vi "cDAQ Channel Tester.vi"(8 "error in (no error)":errorcluster) -> (0 "error out":errorcluster)   [LabVIEW 2016]
uses:
  <resource>/objmgr/daqmx.rc
panel:
  in  "Scan Rate (mSec)":i32=1000
  out "cDAQ Data":string[][](array[string])
  in  "Tab Control":enum32{"Settings"}(tab)
  in  "Tasks In":refnum<k21>[](array[refnum])=["TC Temps-Module 1", "TC Temps-Module 2", "TC Temps-Module 3", "TC Temps-Module 4", "TC Temps-Module 5", "Gas and Temp-Module 6", "AC_DC Events-Module 7"]
  in  "Debug":bool
  out "Debug Data":string[](array[string])
  in  "EXIT":bool
  # "NI DAQ Channel Tester"
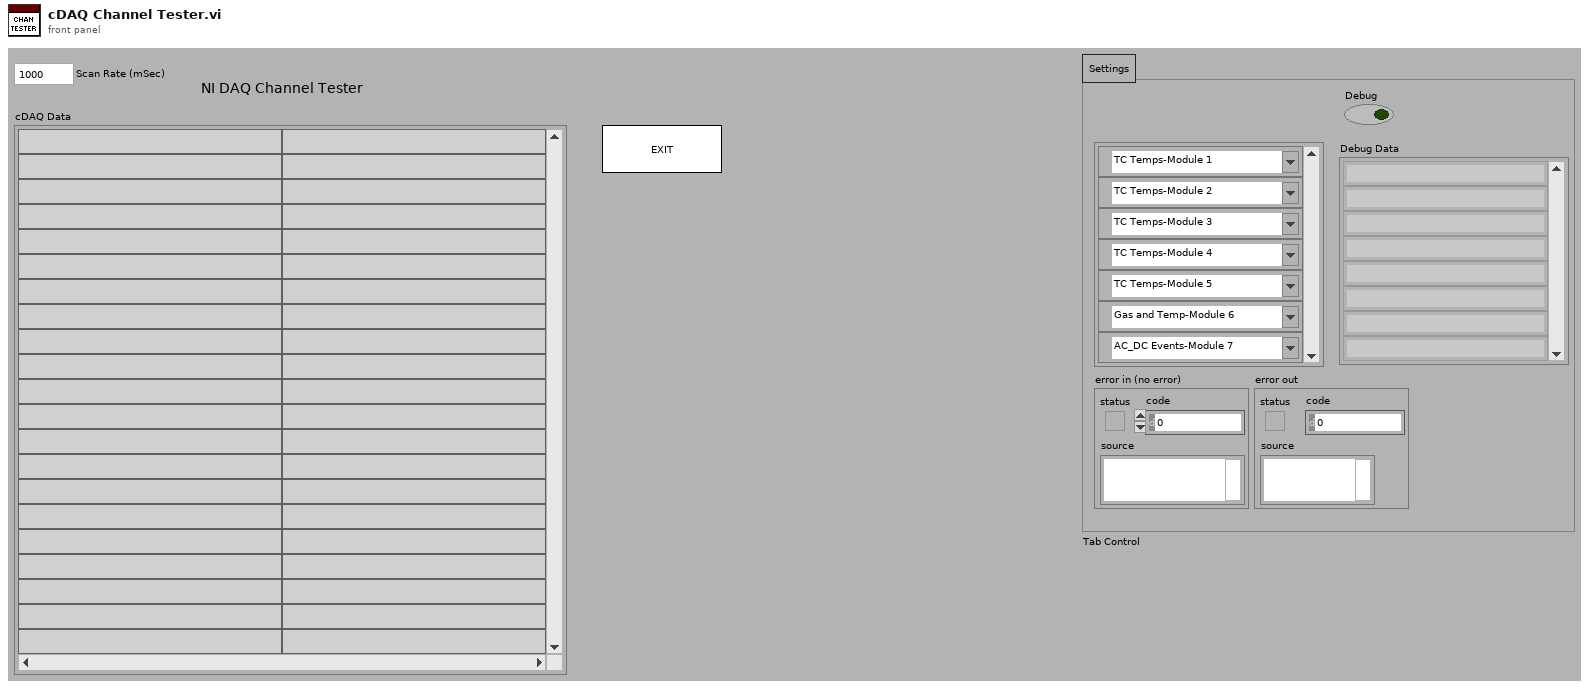
[diagram p1: front panel]
types:
  T1 = enum32{"invalid app kind", "Development System", "Run Time System", "Student Edition", "Embedded LabVIEW", "Evaluation", "Custom"}
  T2 = enum32{"Invalid", "Standard", "Closed", "Hidden", "Minimized", "Maximized"}
  T3 = cluster{"Core":cluster{"Current VI Reference":refnum<vi>, "Close Panel on Exit?":bool}, "Tasks In":refnum<k21>[]}
  T4 = cluster{"Current VI Reference":refnum<vi>, "Close Panel on Exit?":bool}
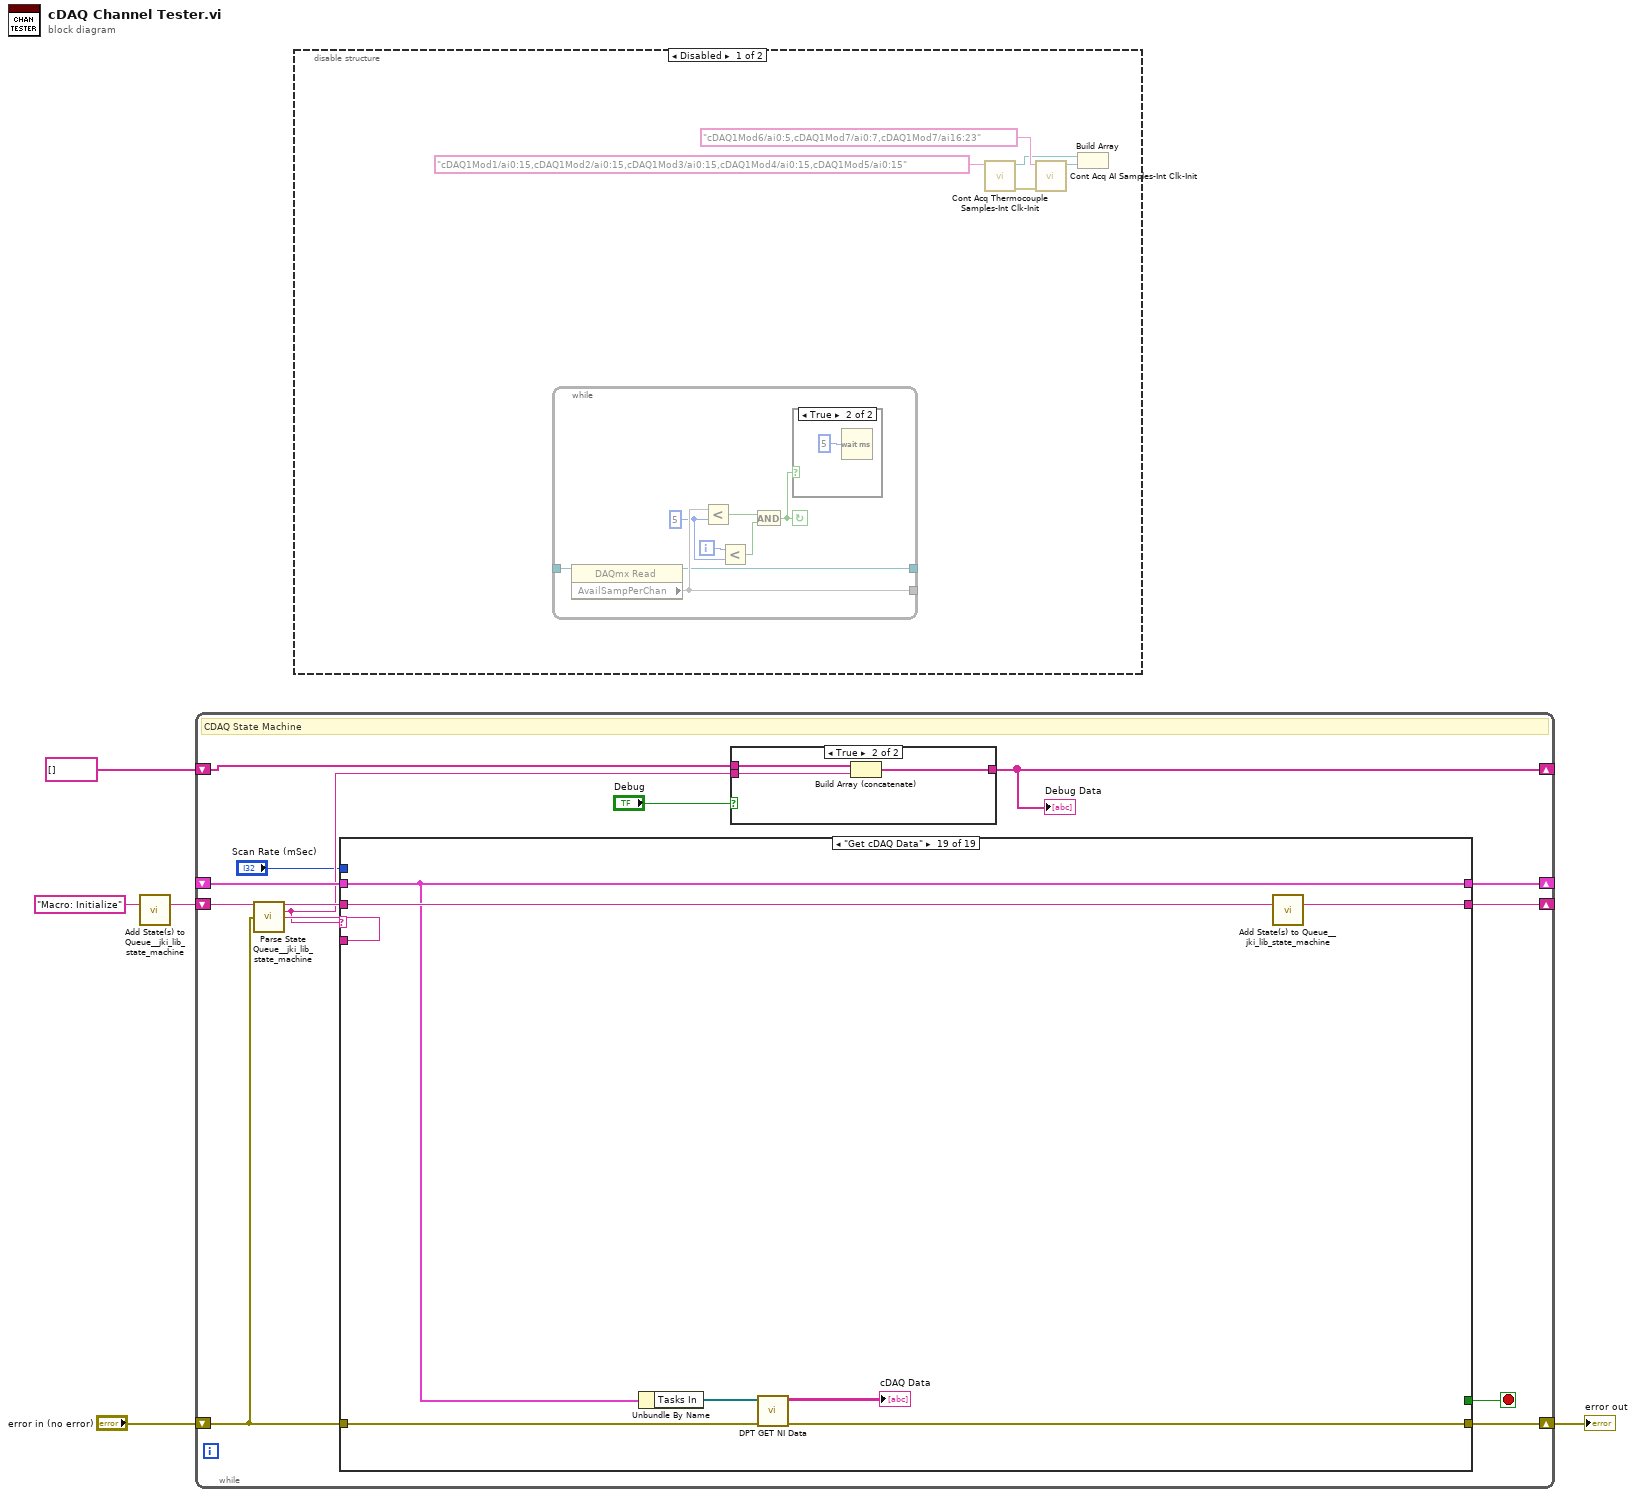
[diagram p0: block diagram]
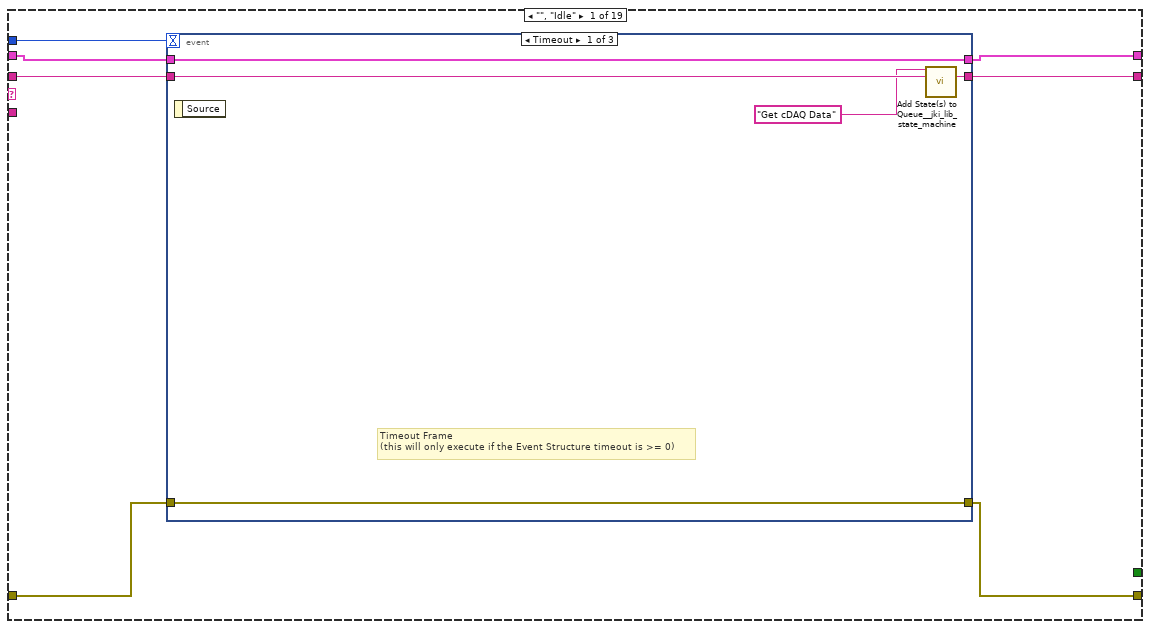
[diagram p5: hidden frame]
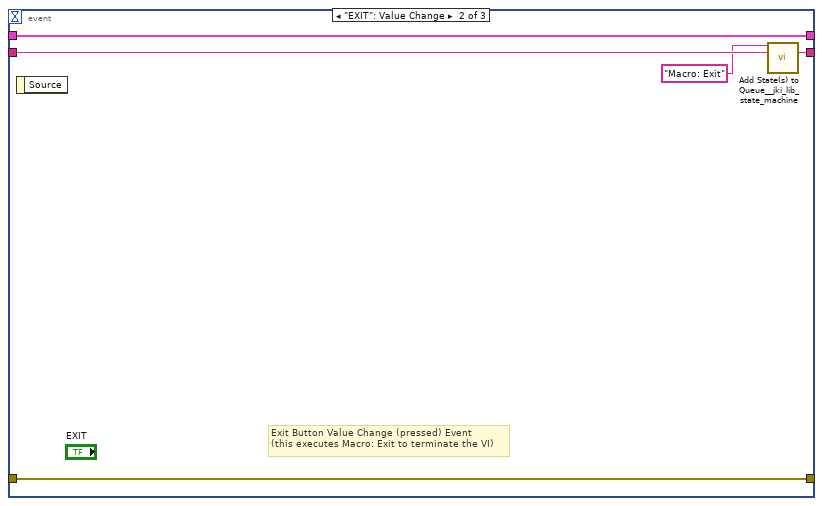
[diagram p6: hidden frame]
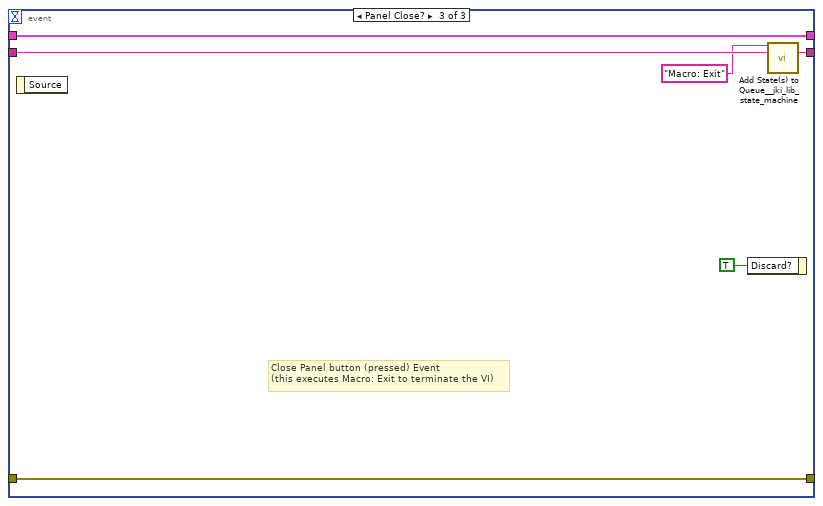
[diagram p7: hidden frame]
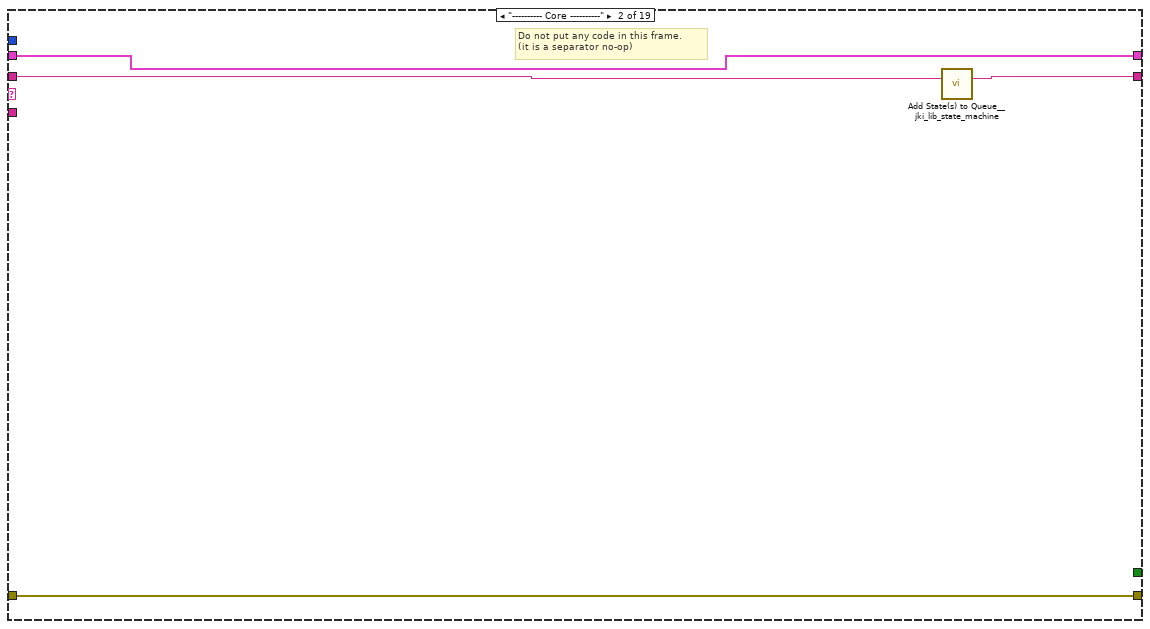
[diagram p8: hidden frame]
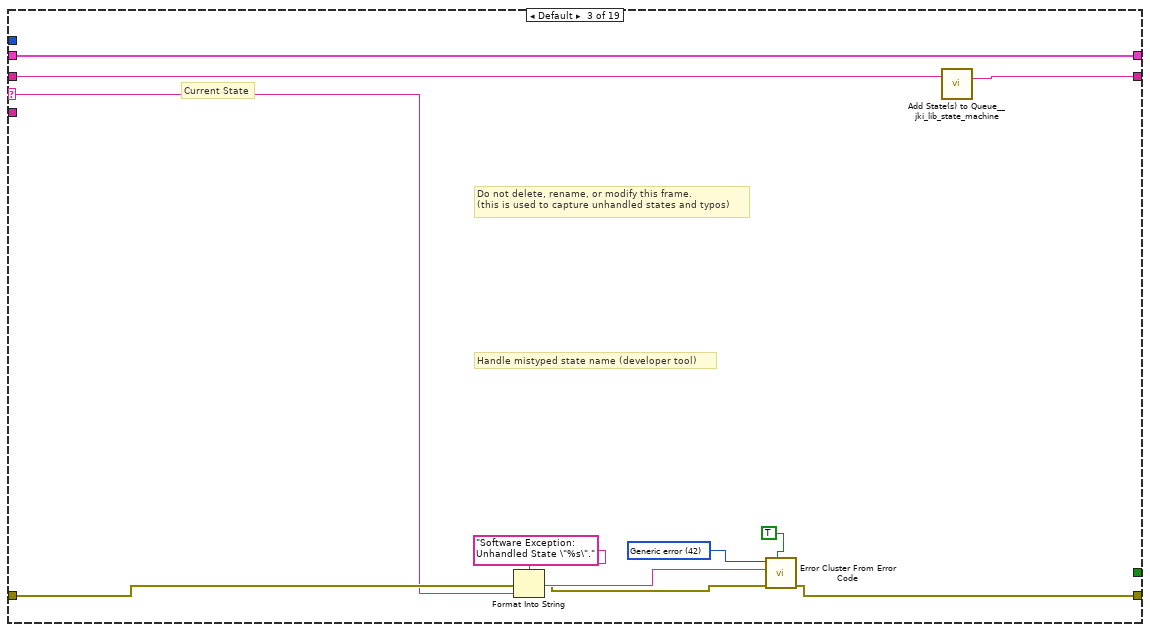
[diagram p9: hidden frame]
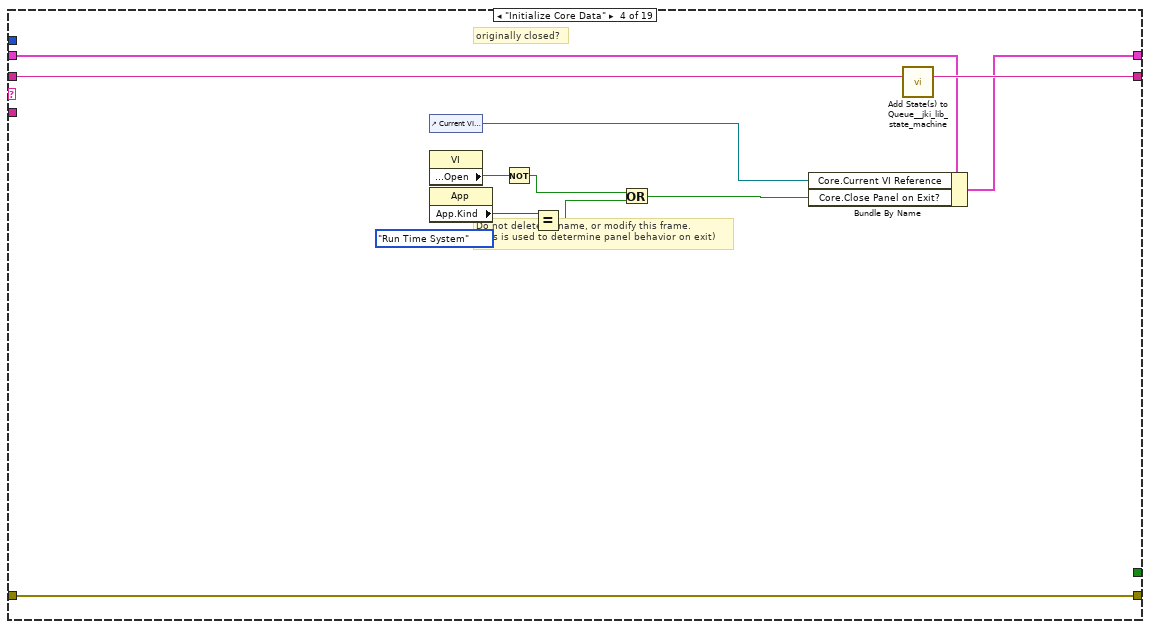
[diagram p10: hidden frame]
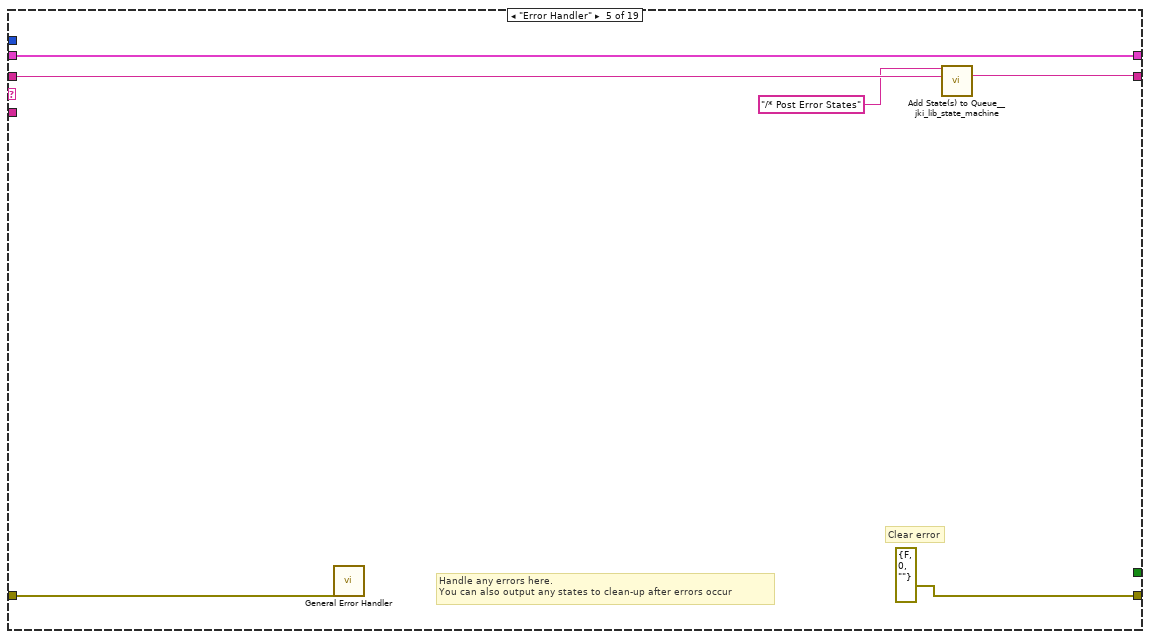
[diagram p11: hidden frame]
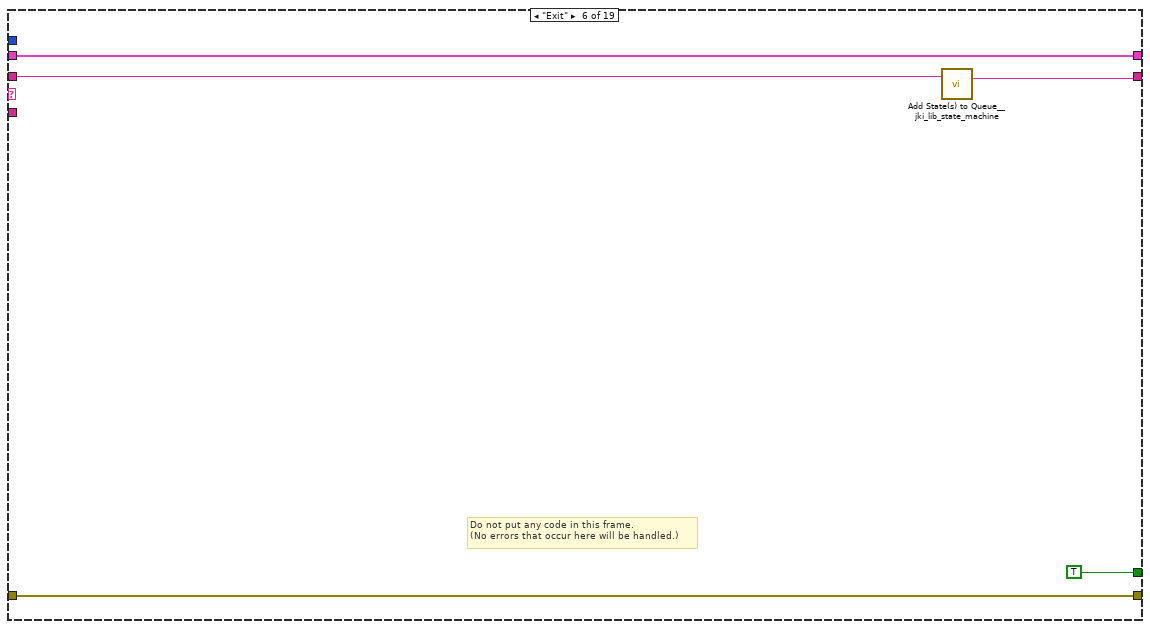
[diagram p12: hidden frame]
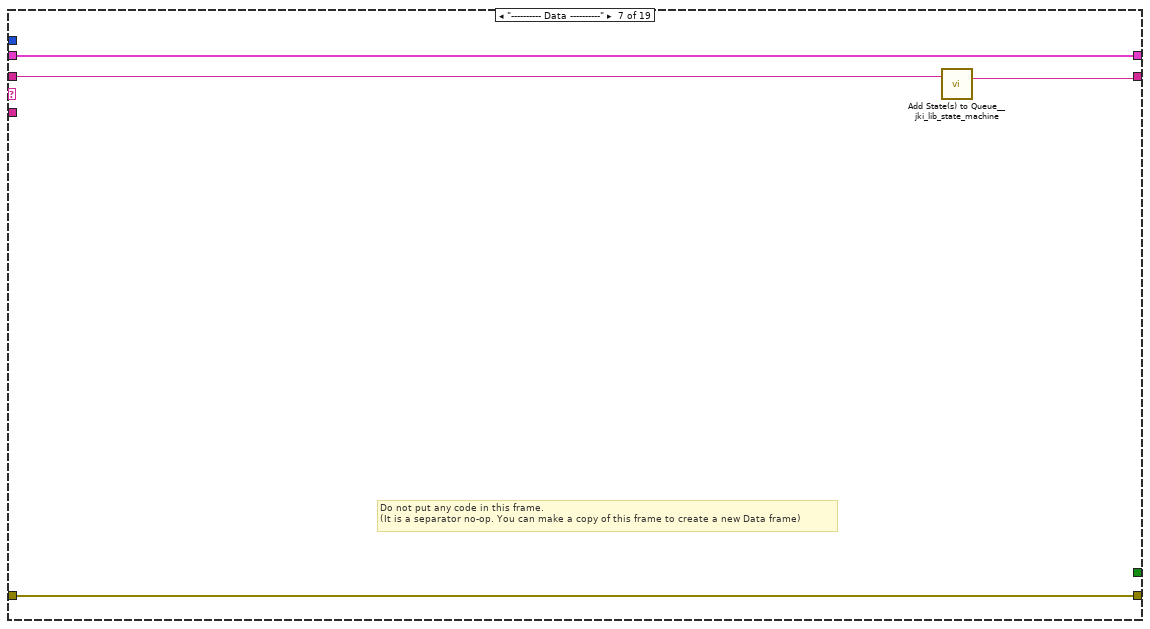
[diagram p13: hidden frame]
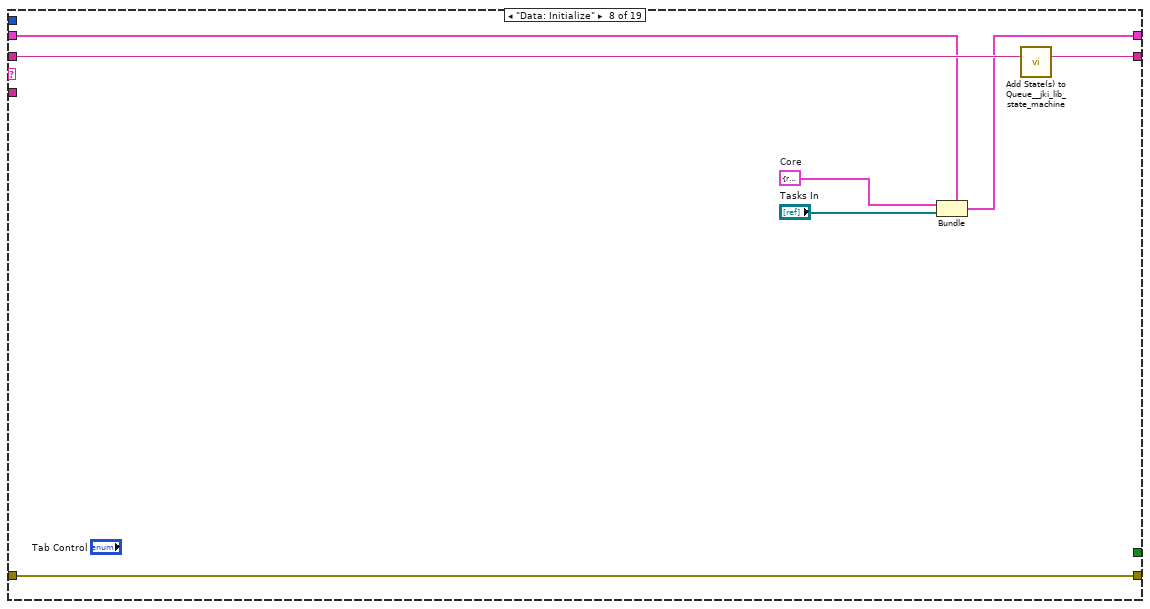
[diagram p14: hidden frame]
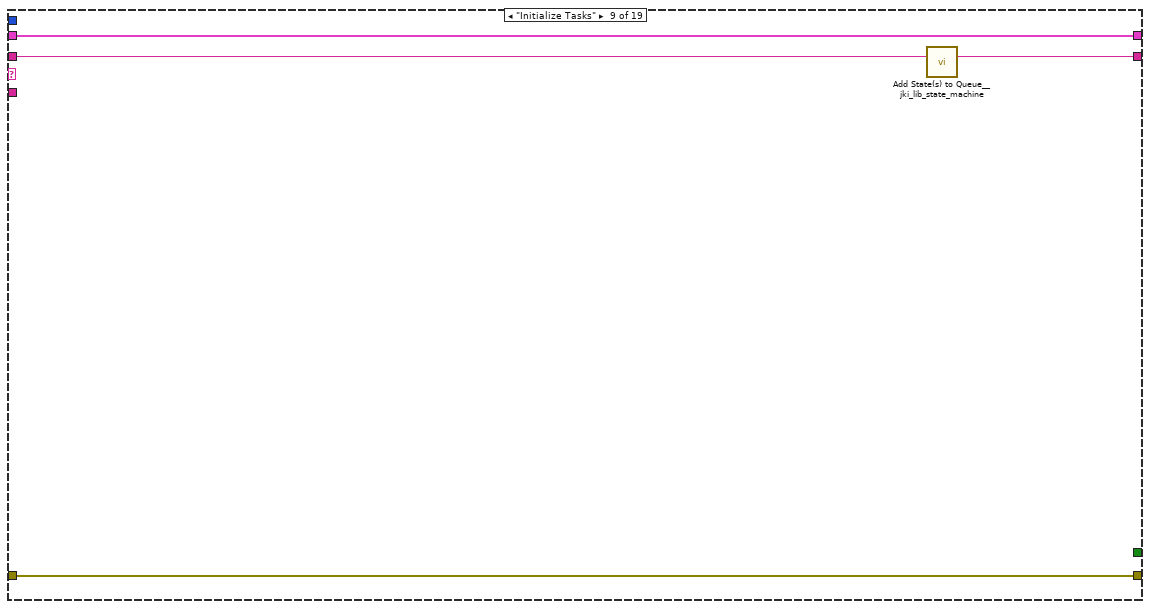
[diagram p15: hidden frame]
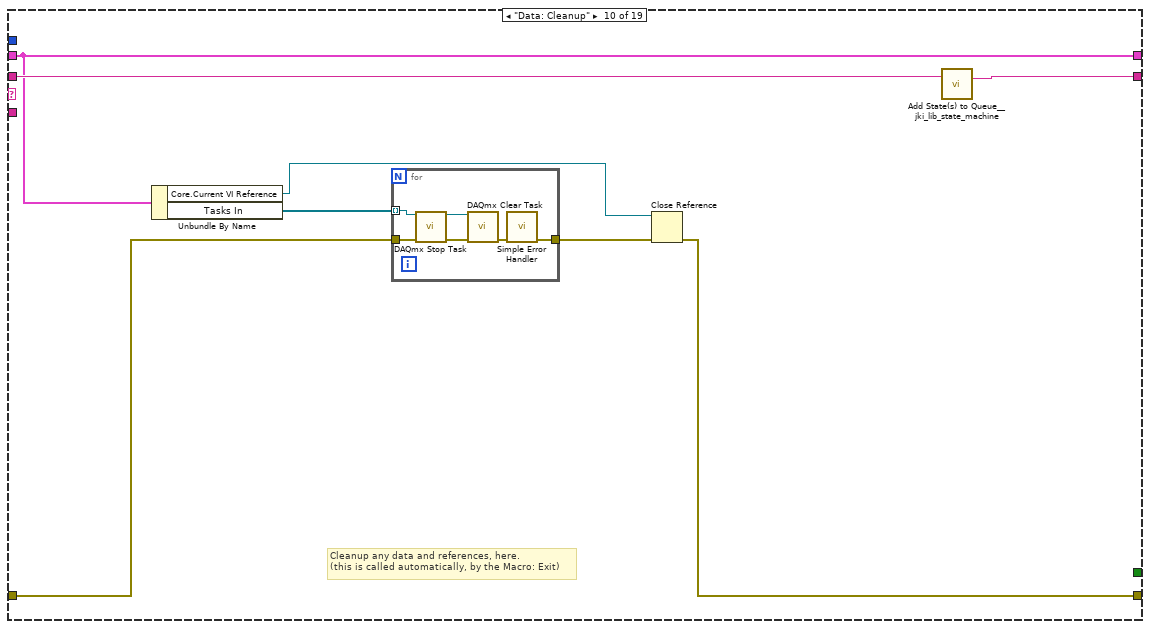
[diagram p16: hidden frame]
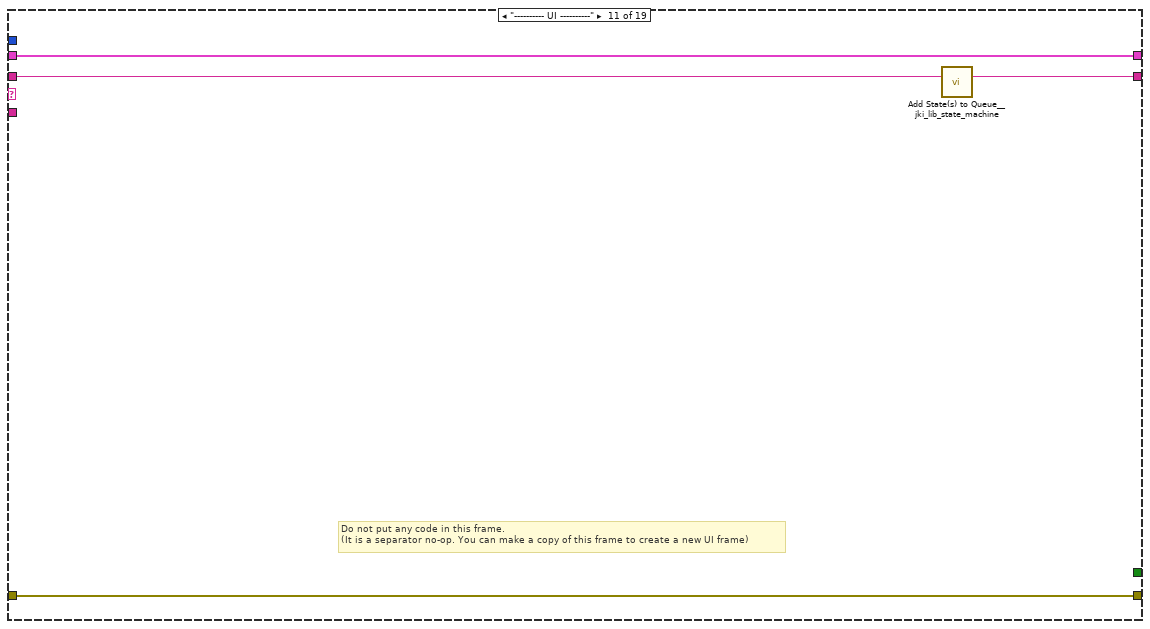
[diagram p17: hidden frame]
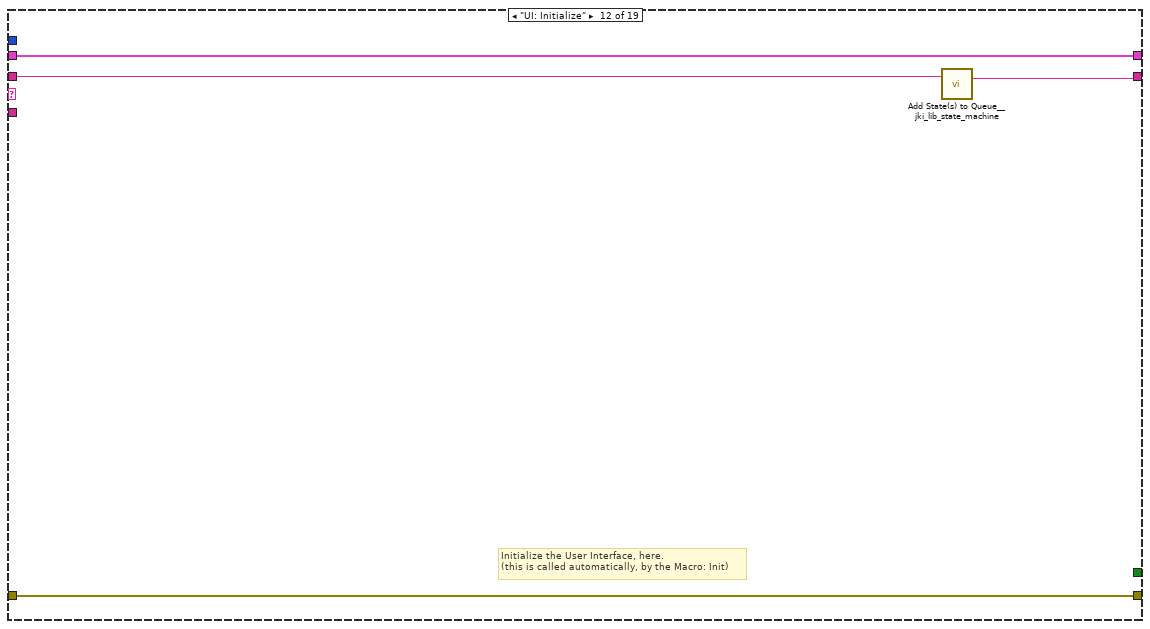
[diagram p18: hidden frame]
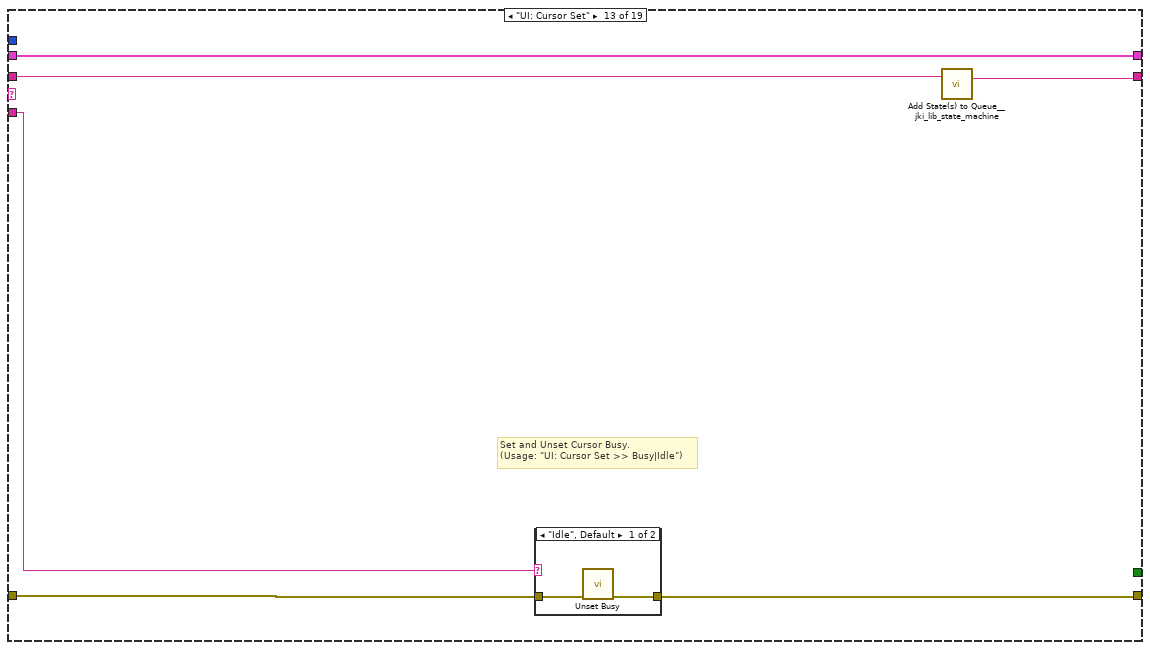
[diagram p19: hidden frame]
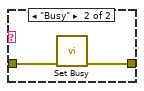
[diagram p20: hidden frame]
diagram:
  n1 = call <vilib>:"Add State(s) to Queue__jki_lib_state_machine.vi"("State(s) in (\"\")"="Macro: Initialize") -> ("States Out"=w5:string)  [unwired: 14 in]
  n2 = while "CDAQ State Machine" {
    shift-right: [w14] -> _
    shift-left: _ -> [w13]
    shift-right: [w16] -> w2
    shift-left: "error in (no error)" -> [w12]
    shift-right: [w15] -> _
    shift-left: w5 -> [w17]
    shift-right: [w9] -> _
    shift-left: string[] [] -> [w10]
    stop <- w11 stop-if-true
    # "CDAQ State Machine"
    n3 = call <vilib>:"Parse State Queue__jki_lib_state_machine.vi"("State Queue"=w17, "Error In (no error)"=w12) -> ("Remaining States"=w19:string, "Current State"=w8:string, "Arguments"=w18:string)  [unwired: 11 in]
    n4 = case shown="\"Get cDAQ Data\"" w8 {
      selector: w8 -> [_ _ w51 _ _ _ _ _ _ _ _ _ _ _ _ _ _ _ _]
      tunnel: w19 -> [w30 w50 w55 w73 w79 w84 w88 w95 w99 w107 w117 w121 w127 w138 w164 w169 w179 w183 w190]
      tunnel: w18 -> [_ _ _ _ _ _ _ _ _ _ _ _ w122 w132 _ _ _ _ _]
      tunnel: w13 -> [w28 w47 w53 w64 w75 w82 w85 w90 w97 w104 w114 w119 w125 w134 w161 w166 w176 w180 w185]
      tunnel: [w27 w48 w57 w70 errorcluster {"status"=FALSE, "code"=0, "source"=""} ("error out") w81 w86 w91 w96 w105 w115 w118 w123 w135 w162 w167 w177 w181 w187] -> w16
      tunnel: w12 -> [w26 w48 w56 w70 w74 w81 w86 w91 w96 w103 w115 w118 w124 w136 w162 w167 w177 w181 w188]
      tunnel: [w29 w49 w54 w72 w78 w83 w87 w94 w98 w106 w116 w120 w126 w137 w163 w168 w178 w182 w189] -> w15
      tunnel: [_ _ _ _ _ TRUE _ _ _ _ _ _ _ _ _ _ _ _ _] -> w11
      tunnel: [w25 w47 w53 w71 w75 w82 w85 w93 w97 w104 w114 w119 w125 w134 w161 w166 w176 w180 w185] -> w14
      tunnel: "Scan Rate (mSec)" -> [w24 _ _ _ _ _ _ _ _ _ _ _ _ _ _ _ _ _ _]
      frame "", "Idle" {
        n5 = event shown="[0] Timeout" {
          selector: _ -> [_ _ _]
          dyn-events: _ -> [_ _ _]
          timeout: w24 -> [_ _ _]
          tunnel: w30 -> [w35 w40 w46]
          tunnel: [w34 w39 w45] -> w29
          tunnel: w28 -> [w32 w37 w43]
          tunnel: [w33 w38 w44] -> w27
          tunnel: w26 -> [w33 w38 w44]
          tunnel: [w32 w37 w43] -> w25
          event Timeout {
            # "Timeout Frame\n(this will only execute if the Event Structure timeout is >= 0)"
            n6 = event-data() -> ()  [unwired: 1 in, 1 out]
            n7 = call <vilib>:"Add State(s) to Queue__jki_lib_state_machine.vi"("State(s) in Front (\"\")"="Get cDAQ Data", "State(s) in (\"\")"=w35) -> ("States Out"=w34:string)  [unwired: 13 in]
          }
          event "EXIT": Value Change {
            # "Exit Button Value Change (pressed) Event\n(this executes Macro: Exit to terminate the VI)"
            n8 = event-data() -> ()  [unwired: 1 in, 1 out]
            n9 = call <vilib>:"Add State(s) to Queue__jki_lib_state_machine.vi"("State(s) in Front (\"\")"="Macro: Exit", "State(s) in (\"\")"=w40) -> ("States Out"=w39:string)  [unwired: 13 in]
          }
          event Panel Close? {
            # "Close Panel button (pressed) Event\n(this executes Macro: Exit to terminate the VI)"
            n10 = event-data() -> ()  [unwired: 1 in, 1 out]
            n11 = event-data("Discard?"=TRUE) -> ()  [unwired: 1 in, 1 out]
            n12 = call <vilib>:"Add State(s) to Queue__jki_lib_state_machine.vi"("State(s) in Front (\"\")"="Macro: Exit", "State(s) in (\"\")"=w46) -> ("States Out"=w45:string)  [unwired: 13 in]
          }
        }
      }
      frame "---------- Core ----------" {
        # "Do not put any code in this frame.\n(it is a separator no-op)"
        n13 = call <vilib>:"Add State(s) to Queue__jki_lib_state_machine.vi"("State(s) in (\"\")"=w50) -> ("States Out"=w49:string)  [unwired: 14 in]
      }
      frame Default {
        w60 = 42 items=["No error", "Argument error", "Memory is full", "Out of zone", "End of file", "File already open", "Generic file I/O error", "File not found", "File permission error", "Disk is full", "Duplicate path", "Too many files open", "System feature not enabled", "Resource file not found", "Cannot add resource", "Resource not found", "Image not found", "Image memory error", "Pen does not exist", "Config type invalid", "Config token not found", "Config parse error", "Config memory error", "Bad external code format", "Bad external code offset", "External code not present", "Null window", "Destroy window error", "Null menu", "Print aborted", "Bad print record", "Print driver error", "Windows error during printing", "Memory error during printing", "Print dialog error", "Generic print error", "Invalid device refnum", "Device not found", "Device parameter error", "Device unit error", "Cannot open device", "Device call aborted", "Generic error", "Cancelled by user", "Object ID too low", "Object ID too high", "Object not in heap", "Unknown heap", "Unknown object (invalid DefProc)", "Unknown object (DefProc not in table)", "Message out of range", "Invalid (null) method", "Unknown message", "Manager call not supported", "Bad address", "Network operation in progress", "Network operation timed out", "Connection is busy", "Network attribute not supported", "Network error", "Address in use", "System out of memory", "Connection aborted", "Connection refused", "Not connected", "Already connected", "Connection closed", "Initialization error (interapplication manager)", "Bad occurrence", "Wait on unbound occurrence handler", "Occurrence queue overflow", "Datalog type conflict", "Unused", "Unrecognized type (interapplication manager)", "Memory corrupt", "Failed to make temporary DLL", "Old CIN version", "Drag socket not found", "Failed to load drop-object", "Failed to register OLE object", "Failed to release OLE object", "Format specifier type mismatch", "Unknown format specifier", "Too few format specifiers", "Too many format specifiers", "Scan failed", "Newer CIN version", "Error converting to variant", "Runtime menu error", "Password tampered", "Variant attribute not found", "Incompatible variant data type", "Event data is not available", "Event Store is not present", "Occurrence is not found", "Event Queue is not created", "Event info is not available", "Refnum passed is NULL", "Error retrieving Class GUID", "Error retrieving CoClass GUID", "Error retrieving TypeLib GUID.", "Bad built application magic bytes.", "Specific driver is different from the specific driver associated with the Logical Name.", "There is no session opened to the class driver.", "Max Error", "MAX - Error with config objects", "MAX - Error loading configuration", "MAX - Group not supported"]
        # "Current State"
        # "Do not delete, rename, or modify this frame.\n(this is used to capture unhandled states and typos)"
        # "Handle mistyped state name (developer tool)"
        n14 = Format Into String(format string="Software Exception: Unhandled State \"%s\"." ("message"), error in=w56, w51) -> (resulting string=w59:string, error out=w58:errorcluster)  [unwired: 1 in]
        n15 = call <vilib>:"Error Cluster From Error Code.vi"("show call chain? (False)"=TRUE, "error in (no error)"=w58, "error message (\"\")"=w59, "error code (0)"=w60) -> ("error out"=w57:errorcluster)  [unwired: 5 in]
        n16 = call <vilib>:"Add State(s) to Queue__jki_lib_state_machine.vi"("State(s) in (\"\")"=w55) -> ("States Out"=w54:string)  [unwired: 14 in]
      }
      frame "Initialize Core Data" {
        # "Do not delete, rename, or modify this frame.\n(this is used to determine panel behavior on exit)"
        # "originally closed?"
        n17 = control-ref of="Current VI Reference"() -> (w62:refnum<vi>)
        n18 = property class="VI"() -> ("Front Panel.Open"=w69:bool)  [unwired: 2 in, 2 out]
        n19 = property class="App"() -> ("App.Kind"=w68:T1)  [unwired: 2 in, 2 out]
        n20 = Not(x=w69) -> (.not. x?=w66:bool)
        n21 = Equal?(x=w68, y=T1."Run Time System" ("Application:Kind")) -> (x = y?=w65:bool)
        n22 = Or(x=w66, y=w65) -> (x .or. y?=w63:bool)
        n23 = Bundle By Name(cluster=w64, "Core.Current VI Reference"=w62, "Core.Close Panel on Exit?"=w63) -> (w71:T3)
        n24 = call <vilib>:"Add State(s) to Queue__jki_lib_state_machine.vi"("State(s) in (\"\")"=w73) -> ("States Out"=w72:string)  [unwired: 14 in]
      }
      frame "Error Handler" {
        # "Handle any errors here.\nYou can also output any states to clean-up after errors occur"
        # "Clear error"
        n25 = call <vilib>:"General Error Handler.vi"("error in (no error)"=w74) -> ()  [unwired: 10 in, 5 out]
        n26 = call <vilib>:"Add State(s) to Queue__jki_lib_state_machine.vi"("State(s) in Front (\"\")"="/* Post Error States", "State(s) in (\"\")"=w79) -> ("States Out"=w78:string)  [unwired: 13 in]
      }
      frame "Exit" {
        # "Do not put any code in this frame.\n(No errors that occur here will be handled.)"
        n27 = call <vilib>:"Add State(s) to Queue__jki_lib_state_machine.vi"("State(s) in (\"\")"=w84) -> ("States Out"=w83:string)  [unwired: 14 in]
      }
      frame "---------- Data ----------" {
        # "Do not put any code in this frame.\n(It is a separator no-op. You can make a copy of this frame to create a new Data frame)"
        n28 = call <vilib>:"Add State(s) to Queue__jki_lib_state_machine.vi"("State(s) in (\"\")"=w88) -> ("States Out"=w87:string)  [unwired: 14 in]
      }
      frame "Data: Initialize" {
        w92 = T4 {"Current VI Reference"=refnum, "Close Panel on Exit?"=FALSE}  # Core
        n29 = Bundle(cluster=w90, "Core"=w92, "Tasks In"="Tasks In") -> (w93:T3)
        n30 = call <vilib>:"Add State(s) to Queue__jki_lib_state_machine.vi"("State(s) in (\"\")"=w95) -> ("States Out"=w94:string)  [unwired: 14 in]
      }
      frame "Initialize Tasks" {
        n31 = call <vilib>:"Add State(s) to Queue__jki_lib_state_machine.vi"("State(s) in (\"\")"=w99) -> ("States Out"=w98:string)  [unwired: 14 in]
      }
      frame "Data: Cleanup" {
        # "Cleanup any data and references, here.\n(this is called automatically, by the Macro: Exit)"
        n32 = Unbundle By Name(w104) -> ("Core.Current VI Reference"=w101:refnum<vi>, "Tasks In"=w100:refnum<k21>[])
        n33 = for {
          tunnel: w103 -> [w112]
          tunnel: [w108] -> w102
          tunnel: w100 -> [w109] mode=indexing
          n34 = call <vilib>:"DAQmx Stop Task.vi"("task/channels in"=w109, "error in"=w112) -> ("task out"=w110:refnum<k21>, "error out"=w111:errorcluster)  [unwired: 12 in]
          n35 = call <vilib>:"DAQmx Clear Task.vi"("task in"=w110, "error in"=w111) -> ("error out"=w113:errorcluster)  [unwired: 13 in]
          n36 = call <vilib>:"Simple Error Handler.vi"("error in (no error)"=w113) -> ("error out"=w108:errorcluster)  [unwired: 4 in, 4 out]
        }
        n37 = Close Reference(reference=w101, error in (no error)=w102) -> (error out=w105:errorcluster)
        n38 = call <vilib>:"Add State(s) to Queue__jki_lib_state_machine.vi"("State(s) in (\"\")"=w107) -> ("States Out"=w106:string)  [unwired: 14 in]
      }
      frame "---------- UI ----------" {
        # "Do not put any code in this frame.\n(It is a separator no-op. You can make a copy of this frame to create a new UI frame)"
        n39 = call <vilib>:"Add State(s) to Queue__jki_lib_state_machine.vi"("State(s) in (\"\")"=w117) -> ("States Out"=w116:string)  [unwired: 14 in]
      }
      frame "UI: Initialize" {
        # "Initialize the User Interface, here.\n(this is called automatically, by the Macro: Init)"
        n40 = call <vilib>:"Add State(s) to Queue__jki_lib_state_machine.vi"("State(s) in (\"\")"=w121) -> ("States Out"=w120:string)  [unwired: 14 in]
      }
      frame "UI: Cursor Set" {
        # "Set and Unset Cursor Busy.\n(Usage: \"UI: Cursor Set >> Busy|Idle\")"
        n41 = case shown="\"Idle\", Default" w122 {
          tunnel: w124 -> [w129 w131]
          tunnel: [w128 w130] -> w123
          frame "Idle", Default {
            n42 = call <vilib>:"Unset Busy.vi"("error in (no error)"=w129) -> ("error out"=w128:errorcluster)  [unwired: 10 in]
          }
          frame "Busy" {
            n43 = call <vilib>:"Set Busy.vi"("error in (no error)"=w131) -> ("error out"=w130:errorcluster)  [unwired: 9 in, 1 out]
          }
        }
        n44 = call <vilib>:"Add State(s) to Queue__jki_lib_state_machine.vi"("State(s) in (\"\")"=w127) -> ("States Out"=w126:string)  [unwired: 14 in]
      }
      frame "UI: Front Panel State" {
        # "Argument"
        # "Set Front Panel Open or Closed\n(Usage: \"UI: Front Panel State >> Open|Close\")"
        n45 = Unbundle By Name(w134) -> ("Core.Current VI Reference"=w133:refnum<vi>)
        n46 = case shown="\"Close\"" w132 {
          tunnel: w136 -> [w142 w155]
          tunnel: [w144 w156] -> w135
          tunnel: w133 -> [w143 w153]
          frame "Open", Default {
            n47 = property class="VI"(reference=w143, error in=w142) -> (reference out=w140:refnum<vi>, error out=w141:errorcluster, "Front Panel.Open"=w139:bool)
            n48 = case shown="False" w139 {
              tunnel: [w147 w150] -> w144
              tunnel: w141 -> [w146 w150]
              tunnel: w140 -> [w145 _]
              frame False {
                n49 = invoke class="VI" method="FP.Open"(reference=w145, error in=w146, "Activate"=TRUE, "State"=T2."Standard") -> (error out=w147:errorcluster)  [unwired: 1 in, 4 out]
              }
              frame True {
              }
            }
          }
          frame "Close" {
            n50 = property class="VI"(reference=w153, error in=w155) -> (reference out=w152:refnum<vi>, error out=w154:errorcluster, "Front Panel.Open"=w151:bool)
            n51 = case shown="True" w151 {
              tunnel: [w157 w160] -> w156
              tunnel: w154 -> [w157 w159]
              tunnel: w152 -> [_ w158]
              frame False {
              }
              frame True {
                n52 = invoke class="VI" method="FP.Close"(reference=w158, error in=w159) -> (error out=w160:errorcluster)  [unwired: 1 in, 2 out]
              }
            }
          }
        }
        n53 = call <vilib>:"Add State(s) to Queue__jki_lib_state_machine.vi"("State(s) in (\"\")"=w138) -> ("States Out"=w137:string)  [unwired: 14 in]
      }
      frame "---------- Macro ----------" {
        # "Do not put any code in this frame.\n(It is a separator no-op. You can make a copy of this frame to create a new Macro frame)"
        n54 = call <vilib>:"Add State(s) to Queue__jki_lib_state_machine.vi"("State(s) in (\"\")"=w164) -> ("States Out"=w163:string)  [unwired: 14 in]
      }
      frame "Macro: Initialize" {
        # "Initialization Macro\n(This is called once, when the VI starts)"
        n55 = call <vilib>:"Add State(s) to Queue__jki_lib_state_machine.vi"("State(s) in Front (\"\")"="Data: Initialize\nInitialize Core Data\nUI: Initialize\nUI: Front Panel State >> Open", "State(s) in (\"\")"=w169) -> ("States Out"=w168:string)  [unwired: 13 in]
      }
      frame "Macro: Exit" {
        # "Exit Macro\n(This is called once, when the VI exits)"
        n56 = Unbundle By Name(w176) -> ("Core.Close Panel on Exit?"=w175:bool)
        n57 = Select(t="UI: Front Panel State >> Close", s=w175, f="") -> (s? t:f=w172:string)
        n58 = call <vilib>:"Add State(s) to Queue__jki_lib_state_machine.vi"("State(s) in (\"\")"=w172, "State(s) at Back (\"\")"="Data: Cleanup\nExit") -> ("States Out"=w170:string)  [unwired: 13 in]
        n59 = call <vilib>:"Add State(s) to Queue__jki_lib_state_machine.vi"("State(s) in Front (\"\")"=w170, "State(s) in (\"\")"=w179) -> ("States Out"=w178:string)  [unwired: 13 in]
      }
      frame "------ TestDAQ ------" {
        # "Template Separator\n(You can make a copy of, or modify, this frame)"
        n60 = call <vilib>:"Add State(s) to Queue__jki_lib_state_machine.vi"("State(s) in (\"\")"=w183) -> ("States Out"=w182:string)  [unwired: 14 in]
      }
      frame "Get cDAQ Data" {
        n61 = Unbundle By Name(w185) -> ("Tasks In"=w184:refnum<k21>[])
        n62 = call "DPT GET NI Data.vi"("error in (no error)"=w188, "Tasks In"=w184) -> ("error out"=w187:errorcluster, "cDAQ Data"=→"cDAQ Data":string[][])  [unwired: 7 in, 1 out]
        n63 = call <vilib>:"Add State(s) to Queue__jki_lib_state_machine.vi"("State(s) in (\"\")"=w190) -> ("States Out"=w189:string)  [unwired: 14 in]
      }
    }
    n64 = case shown="True" "Debug" {
      tunnel: w10 -> [w20 w23]
      tunnel: [w20 w22] -> w9
      tunnel: w8 -> [_ w21]
      frame False {
      }
      frame True {
        n65 = Build Array (concatenate)(w23, w21) -> (w22:string[])
      }
    }
    "Debug Data" <- w9
  }
  "error out" <- w2
  n66 = disable-structure shown="Disabled" {
    frame Disabled {
      n67 = while {
        tunnel: _ -> [w203]
        tunnel: [w201] -> _
        tunnel: [w198] -> _
        i -> [w196]
        stop <- w197 continue-if-true
        w200 = u32 5 ("y")
        n68 = property class="DAQmx Read"(reference=w203) -> (reference out=w198:refnum<k21>, "AvailSampPerChan"=w201)  [unwired: 1 in, 1 out]
        n69 = Less?(x=w201, y=w200) -> (x < y?=w202:bool)
        n70 = Less?(x=w196, y=w200) -> (x < y?=w199:bool)
        n71 = And(x=w202, y=w199) -> (x .and. y?=w197:bool)
        n72 = case shown="True" w197 {
          frame False {
          }
          frame True {
            n73 = Wait (ms)(milliseconds to wait=u32 5) -> ()  [unwired: 1 out]
          }
        }
      }
      n74 = call "Cont Acq Thermocouple Samples-Int Clk-Init.vi"("Physical Channel"="cDAQ1Mod1/ai0:15,cDAQ1Mod2/ai0:15,cDAQ1Mod3/ai0:15,cDAQ1Mod4/ai0:15,cDAQ1Mod5/ai0:15" ("name to assign")) -> ("Temp task out"=w193:refnum<k21>, "error out"=w191:errorcluster)  [unwired: 8 in]
      n75 = call "Cont Acq AI Samples-Int Clk-Init.vi"("error in"=w191, "physical channels"="cDAQ1Mod6/ai0:5,cDAQ1Mod7/ai0:7,cDAQ1Mod7/ai16:23" ("name to assign")) -> ("AI task out"=w192:refnum<k21>)  [unwired: 8 in, 1 out]
      n76 = Build Array(w193, w192) -> ()  [unwired: 1 out]
    }
    frame Enabled {
    }
  }
